vi "Set DC Voltage Offset.vi"(8 "error in (no error)":errorcluster, 10 "Offset Value (0.0)":dbl format="%^.3e", 11 "VISA resource name":refnum<visa-resource-name>) -> (0 "error out":errorcluster, 3 "VISA resource name out":refnum<visa-resource-name>)   [LabVIEW 2013, in "Fluke 5XXX Series Multicalibrators.lvlib"]
doc: "This VI applies a dc offset to an ac output voltage (maximum six digits). This VI applies only to single ac voltage outputs. If the selected offset is too large for the active ac voltage range, an error message is returned.\n\nNote:\n\nThis VI is available only for instrument models 5500A and 5520A."
uses:
  Fluke 5XXX Series Multicalibrators.lvlib
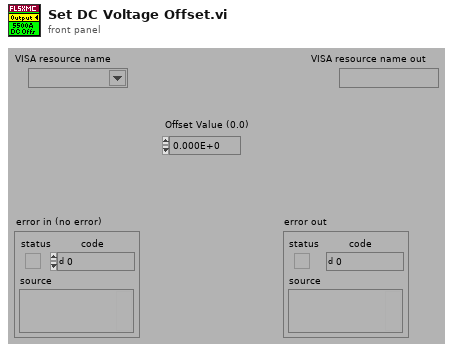
[diagram p1: front panel]
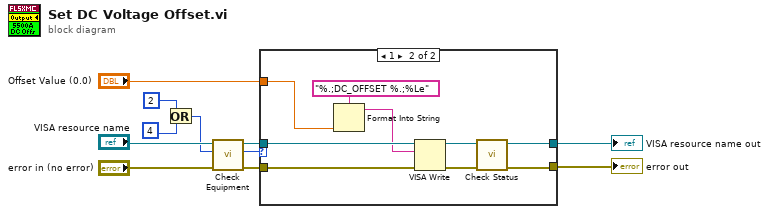
[diagram p0: block diagram]
diagram:
  n1 = Or(x=2 ("Numeric"), y=4 ("Numeric")) -> (x .or. y?=w3:i32)
  n2 = call "Check Equipment.vi"("error in (no error)"="error in (no error)", "Bit Mask"=w3, "VISA resource name"="VISA resource name") -> ("error out"=w11:errorcluster, "Present?"=w10:u32, "VISA resource name out"=w9:refnum<visa-resource-name>)  [unwired: 6 in]
  n3 = case shown="1" w10 {
    tunnel: "Offset Value (0.0)" -> [_ w14]
    tunnel: [w12 w17] -> w8
    tunnel: w11 -> [w13 w22]
    tunnel: w9 -> [w12 w21]
    tunnel: [w13 w20] -> w7
    frame 0, Default {
    }
    frame 1 {
      n4 = Format Into String(format string="%.;DC_OFFSET %.;%Le", w14) -> (resulting string=w15:string)  [unwired: 2 in, 1 out]
      n5 = VISA Write(VISA resource name=w21, write buffer=w15, error in (no error)=w22) -> (VISA resource name out=w18:refnum<visa-resource-name>, error out=w19:errorcluster)  [unwired: 1 out]
      n6 = call "Check Status.vi"("VISA resource name"=w18, "error in (no error)"=w19) -> ("VISA resource name out"=w17:refnum<visa-resource-name>, "error out"=w20:errorcluster)  [unwired: 12 in]
    }
  }
  "VISA resource name out" <- w8
  "error out" <- w7
